vi "Begin.vi"(11 "Image Size":T1=enum."160x120") -> (0 "error out":errorcluster)   [LabVIEW 2012]
doc: "Called before other user functions, this VI is expected to open initial I/O refnums, load in file data, and do all program initialization. Notice that the <B>error out</B> terminal is simply used for data flow. Wiring it to other structures or subVIs ensures that this VI runs first."
uses:
  <vilib>/Rock Robotics/WPI/Camera/WPI_CameraImageSize.ctl
  <vilib>/Rock Robotics/WPI/Camera/WPI_CameraWhite Balance Values.ctl
  <vilib>/Rock Robotics/WPI/Camera/WPI_CameraExposure Values.ctl
  <vilib>/Rock Robotics/WPI/Camera/WPI_CameraFrameRate.ctl
  <vilib>/Rock Robotics/WPI/DriverStation/WPI_DriverStationRobotMode2.ctl
  <vilib>/Rock Robotics/WPI/Joystick/WPI_JoystickDeviceEnum.ctl
  <vilib>/Rock Robotics/SystemInterfaces/DIO/FPGA_DIORelayChannel.ctl
  <vilib>/Rock Robotics/WPI/Relay/WPI_RelayDirection.ctl
  <vilib>/Rock Robotics/SystemInterfaces/DIO/FPGA_DIOChannel.ctl
  <vilib>/Rock Robotics/WPI/Solenoid/WPI_SolenoidChannel.ctl
  <vilib>/Rock Robotics/WPI/Relay/WPI_RelayValue.ctl
  <vilib>/Rock Robotics/SystemInterfaces/DIO/FPGA_DIOPWMChannel.ctl
  <vilib>/Rock Robotics/WPI/SafetyOutput/WPI_SafetyOutputConfigMenu.ctl
  <vilib>/Rock Robotics/SystemInterfaces/AI/FPGA_AIGyroChannel.ctl
  <vilib>/Rock Robotics/SystemInterfaces/AI/FPGA_AIChannel.ctl
  Robot Global Data.vi
  <vilib>/Rock Robotics/WPI/Solenoid/WPI_SolenoidOpenSingle.vi
  <vilib>/Rock Robotics/WPI/MotorControl/WPI_MotorControlOpen Victor.vi
  <vilib>/Rock Robotics/WPI/MotorControl/WPI_MotorControlOpen Jaguar.vi
  <vilib>/Rock Robotics/WPI/RobotDrive/WPI_RobotDriveOpen4MotorWithVictor.vi
  <vilib>/Rock Robotics/WPI/Compressor/WPI_CompressorGetSetRefNum.vi
  <vilib>/Rock Robotics/WPI/RobotDrive/WPI_RobotDriveOpen2MotorWithTalon.vi
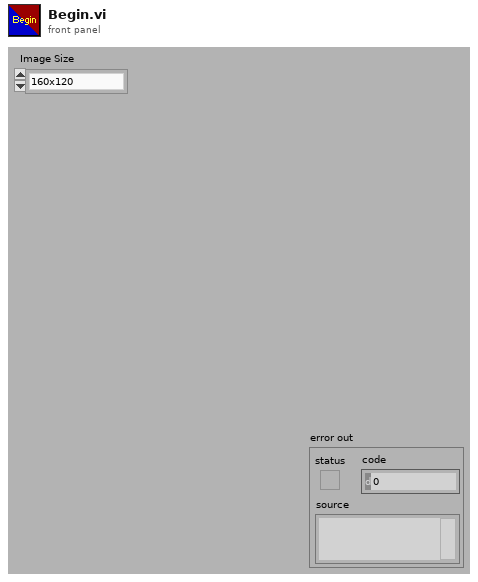
[diagram p1: front panel]
types:
  T1 = typedef "WPI_CameraImageSize.ctl" = enum16{"640x480", "320x240", "160x120"}
  T2 = typedef "WPI_SafetyOutputConfigMenu.ctl" = enum16{"Enable", "Disable"}
  T3 = typedef "WPI_SolenoidChannel.ctl" = enum8{"Solenoid 1", "Solenoid 2", "Solenoid 3", "Solenoid 4", "Solenoid 5", "Solenoid 6", "Solenoid 7", "Solenoid 8", "Invalid"}
  T4 = typedef "FPGA_AIChannel.ctl" = enum8{"AI 1", "AI 2", "AI 3", "AI 4", "AI 5", "AI 6", "AI 7", "AI 8", "Invalid"}
  T5 = typedef "FPGA_DIOPWMChannel.ctl" = enum8{"PWM 1", "PWM 2", "PWM 3", "PWM 4", "PWM 5", "PWM 6", "PWM 7", "PWM 8", "PWM 9", "PWM 10", "Invalid"}
  T6 = typedef "FPGA_AIGyroChannel.ctl" = enum8{"AI 1", "AI 2", "Invalid"}
  T7 = typedef "FPGA_DIOChannel.ctl" = enum8{"DIO 1", "DIO 2", "DIO 3", "DIO 4", "DIO 5", "DIO 6", "DIO 7", "DIO 8", "DIO 9", "DIO 10", "DIO 11", "DIO 12", "DIO 13", "DIO 14", "Invalid"}
  T8 = typedef "WPI_JoystickDeviceEnum.ctl" = enum16{"USB 1", "USB 2", "USB 3", "USB 4", "Kinect 1", "Kinect 2"}
  T9 = typedef "WPI_RelayValue.ctl" = enum16{"Off", "On", "Forward", "Reverse"}
  T10 = typedef "FPGA_DIORelayChannel.ctl" = enum8{"Relay 1", "Relay 2", "Relay 3", "Relay 4", "Relay 5", "Relay 6", "Relay 7", "Relay 8", "Invalid"}
  T11 = typedef "WPI_RelayDirection.ctl" = enum16{"Both directions", "Forward only", "Reverse only"}
  T12 = typedef "WPI_DriverStationRobotMode2.ctl" = enum16{"Autonomous Disabled", "Autonomous Enabled", "Teleop Disabled", "Teleop Enabled", "Timeout", "Finish", "Test Disabled", "Test Enabled"}
  T13 = typedef "WPI_CameraFrameRate.ctl" = u32
  T14 = typedef "WPI_CameraExposure Values.ctl" = enum16{"Auto", "Flicker-free 50 Hz", "Flicker-free 60 Hz", "Hold current"}
  T15 = typedef "WPI_CameraWhite Balance Values.ctl" = enum16{"Auto", "Fixed indoor", "Fixed outdoor 1", "Fixed outdoor 2", "Fixed fluorescent 1", "Fixed fluorescent 2", "Hold current"}
  T16 = typedef "WPI_RobotDriveDevRef.ctl" = cluster{"DevStatus":errorcluster, "Motors[]":T17[], "Square Inputs":bool, "Max Output":dbl, "Isochronous":bool}
  T17 = typedef "WPI_MotorControlDeviceRef.ctl" = cluster{"DeviceStatus":errorcluster, "Type":enum16{"PWM", "CAN"}, "PWM":cluster{"Digital Module":T18, "PWM Channel":T5, "DeadBand":T19}, "CAN":cluster{"Device Number":u8, "Control Mode":T20, "Semaphore":T21, "Max Vout":dbl}, "Invert":bool, "TransformRef":T22, "InvTransformRef":T22}
  T18 = typedef "FPGA_TypedefDigitalModule.ctl" = enum16{"Digital Module 1", "Digital Module 2"}
  T19 = typedef "WPI_PWMDeadband.ctl" = cluster{"Name":string, "maxPositivePwm":i32, "minPositivePwm":i32, "centerPwm":i32, "maxNegativePwm":i32, "minNegativePwm":i32, "angularRange":u16}
  T20 = typedef "WPI_CANJaguar_ControlMode.ctl" = enum8{"Percent VBus", "Current", "Speed", "Position", "Voltage"}
  T21 = typedef "Semaphore RefNum" = refnum<k1>
  T22 = typedef "WPI_PWMTransform_ConPane.ctl" = refnum<vi>
  T23 = typedef "WPI_SolenoidDevRef.ctl" = cluster{"DevStatus":errorcluster, "Solenoid Module":T24, "Forward Solenoid Channel":T3, "Reverse Solenoid Channel":T3}
  T24 = typedef "FPGA_TypedefSolenoidModule.ctl" = enum16{"Solenoid Module 1", "Solenoid Module 2"}
  T25 = typedef "WPI_JoystickDevRef.ctl" = cluster{"Device":T8}
  T26 = typedef "WPI_CameraDevRef.ctl" = cluster{"Camera Address":string, "CameraStatus":errorcluster, "Acquire Image Notifier":refnum<notifier>}
  T27 = typedef "WPI_RelayDevRef.ctl" = cluster{"DevStatus":errorcluster, "Relay Channel":T10, "Digital Module":T18, "Relay Direction":T11}
  T28 = typedef "WPI_GyroDevRef.ctl" = cluster{"DevStatus":errorcluster, "Analog Module":T29, "Analog Channel":T4, "Offset":dbl, "Gain (VoltsPerDegree/Second)":dbl}
  T29 = typedef "FPGA_TypedefAnalogModule.ctl" = enum16{"Analog Module 1", "Analog Module 2"}
  T30 = typedef "WPI_CompressorDevRef.ctl" = cluster{"DevStatus":errorcluster, "DigitalInputDevRef":T31, "RelayDevRef":T27}
  T31 = typedef "WPI_DigitalInputDevRef.ctl" = cluster{"DevStatus":errorcluster, "DIO Channel":T7, "Digital Module":T18}
  T32 = typedef "WPI_AnalogChannelDevRef.ctl" = cluster{"DevStatus":errorcluster, "Analog Module":T29, "Analog Channel":T4}
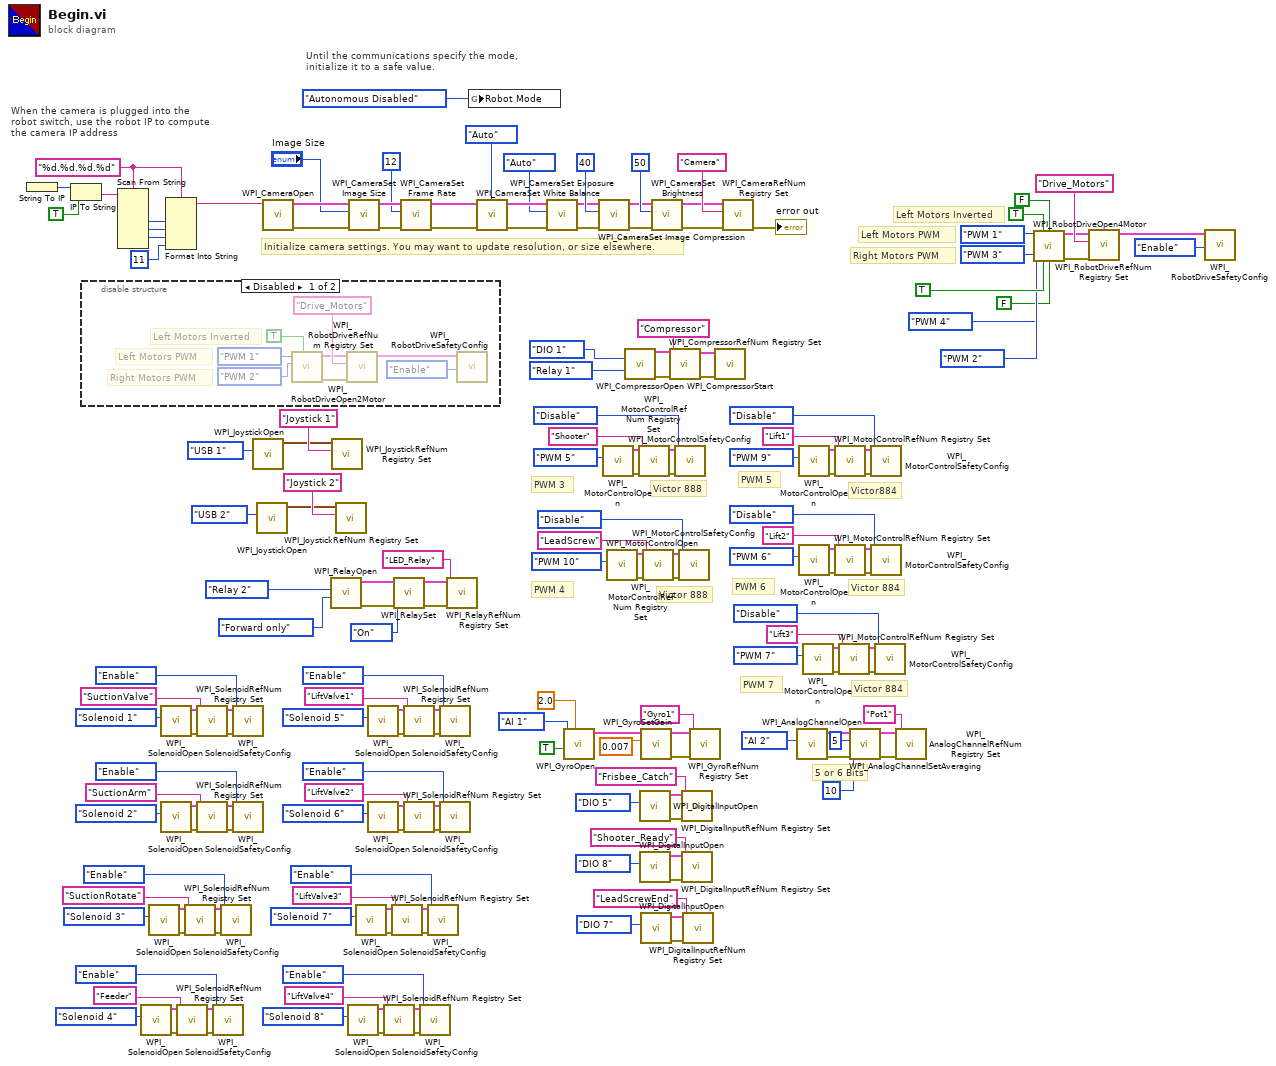
[diagram p0: block diagram]
diagram:
  w38 = "%d.%d.%d.%d" ("format string")
  # "5 or 6 Bits"
  # "PWM 7"
  # "PWM 6"
  # "PWM 5"
  # "PWM 3"
  # "PWM 4"
  # "Right Motors PWM"
  # "Left Motors PWM"
  # "Left Motors Inverted"
  # "Victor884"
  # "Victor 884"
  # "Victor 884"
  # "Victor 888"
  # "Victor 888"
  # "Until the communications specify the mode,\ninitialize it to a safe value."
  # "When the camera is plugged into the\nrobot switch, use the robot IP to compute\nthe camera IP address"
  # "Initialize camera settings. You may want to update resolution, or size elsewhere."
  n1 = String To IP() -> (0:w164:u32)  [unwired: 1 in]
  n2 = IP To String(1:TRUE ("dot notation? (F)"), 2:w164) -> (0:w162:string)
  n3 = disable-structure shown="Disabled" {
    frame Disabled {
      # "Right Motors PWM"
      # "Left Motors PWM"
      # "Left Motors Inverted"
      n4 = call-poly <vilib>:"WPI_RobotDriveOpen2Motor.vi"("Left Motor Inverted"=TRUE, "Right Motor"=FPGA_DIOPWMChannel."PWM 2", "Left Motor"=FPGA_DIOPWMChannel."PWM 1") -> ("error out"=w190:errorcluster, "RobotDriveDevRef"=w189:T16)  [unwired: 7 in]
      n5 = call <vilib>:"WPI_RobotDriveRefNum Registry Set.vi"("error in (no error)"=w190, "refnum name"="Drive_Motors", "RobotDriveDevRef"=w189) -> ("RobotDriveDevRef"=w192:T16)  [unwired: 8 out]
      n6 = call <vilib>:"WPI_RobotDriveSafetyConfig.vi"("mode"=WPI_SafetyOutputConfigMenu."Enable", "RobotDriveDevRef"=w192) -> ()  [unwired: 8 in, 2 out]
    }
    frame Enabled {
    }
  }
  n7 = Scan From String(format string=w38, input string=w162) -> (output 1=w161:i32, output 2=w160:i32, output 3=w159:i32)  [unwired: 7 in, 3 out]
  n8 = call-poly <vilib>:"WPI_SolenoidOpen.vi"("Solenoid Channel"=WPI_SolenoidChannel."Solenoid 4") -> ("error out"=w71:errorcluster, "SolenoidDevRef"=w72:T23)  [unwired: 9 in]
  n9 = call-poly <vilib>:"WPI_SolenoidOpen.vi"("Solenoid Channel"=WPI_SolenoidChannel."Solenoid 3") -> ("error out"=w82:errorcluster, "SolenoidDevRef"=w83:T23)  [unwired: 9 in]
  n10 = call-poly <vilib>:"WPI_SolenoidOpen.vi"("Solenoid Channel"=WPI_SolenoidChannel."Solenoid 1") -> ("error out"=w140:errorcluster, "SolenoidDevRef"=w141:T23)  [unwired: 9 in]
  n11 = call-poly <vilib>:"WPI_SolenoidOpen.vi"("Solenoid Channel"=WPI_SolenoidChannel."Solenoid 2") -> ("error out"=w103:errorcluster, "SolenoidDevRef"=w104:T23)  [unwired: 9 in]
  n12 = Format Into String(format string=w38, w161, w160, w159, 11 ("Compression")) -> (resulting string=w156:string)  [unwired: 2 in, 1 out]
  n13 = call <vilib>:"WPI_SolenoidRefNum Registry Set.vi"("error in (no error)"=w71, "refnum name"="Feeder", "SolenoidDevRef"=w72) -> ("error out"=w68:errorcluster, "SolenoidDevRef"=w67:T23)  [unwired: 7 in]
  n14 = call <vilib>:"WPI_SolenoidRefNum Registry Set.vi"("error in (no error)"=w82, "refnum name"="SuctionRotate", "SolenoidDevRef"=w83) -> ("error out"=w79:errorcluster, "SolenoidDevRef"=w78:T23)  [unwired: 7 in]
  n15 = call <vilib>:"WPI_SolenoidRefNum Registry Set.vi"("error in (no error)"=w140, "refnum name"="SuctionValve", "SolenoidDevRef"=w141) -> ("error out"=w126:errorcluster, "SolenoidDevRef"=w125:T23)  [unwired: 7 in]
  n16 = call <vilib>:"WPI_SolenoidRefNum Registry Set.vi"("error in (no error)"=w103, "refnum name"="SuctionArm", "SolenoidDevRef"=w104) -> ("error out"=w100:errorcluster, "SolenoidDevRef"=w99:T23)  [unwired: 7 in]
  n17 = call <vilib>:"WPI_SolenoidSafetyConfig.vi"("error in (no error)"=w68, "mode"=WPI_SafetyOutputConfigMenu."Enable", "SolenoidDevRef"=w67) -> ()  [unwired: 7 in, 2 out]
  n18 = call <vilib>:"WPI_SolenoidSafetyConfig.vi"("error in (no error)"=w79, "mode"=WPI_SafetyOutputConfigMenu."Enable", "SolenoidDevRef"=w78) -> ()  [unwired: 7 in, 2 out]
  n19 = call <vilib>:"WPI_SolenoidSafetyConfig.vi"("error in (no error)"=w126, "mode"=WPI_SafetyOutputConfigMenu."Enable", "SolenoidDevRef"=w125) -> ()  [unwired: 7 in, 2 out]
  n20 = call <vilib>:"WPI_SolenoidSafetyConfig.vi"("error in (no error)"=w100, "mode"=WPI_SafetyOutputConfigMenu."Enable", "SolenoidDevRef"=w99) -> ()  [unwired: 7 in, 2 out]
  n21 = call <vilib>:"WPI_JoystickOpen.vi"("JoystickDevice"=WPI_JoystickDeviceEnum."USB 1") -> ("JoystickDevRef"=w154:T25)  [unwired: 10 in]
  n22 = call <vilib>:"WPI_JoystickOpen.vi"("JoystickDevice"=WPI_JoystickDeviceEnum."USB 2") -> ("JoystickDevRef"=w64:T25)  [unwired: 10 in]
  n23 = call <vilib>:"WPI_CameraOpen.vi"("Camera Address"=w156) -> ("error out"=w176:errorcluster, "CameraDevRef"=w177:T26)  [unwired: 1 in, 8 out]
  n24 = call <vilib>:"WPI_RelayOpen.vi"("Relay Direction"=WPI_RelayDirection."Forward only", "Relay Channel"=FPGA_DIORelayChannel."Relay 2") -> ("error out"=w137:errorcluster, "RelayDevRef"=w136:T27)  [unwired: 8 in]
  n25 = call <vilib>:"WPI_JoystickRefNum Registry Set.vi"("refnum name"="Joystick 1", "JoystickDevRef"=w154) -> ()  [unwired: 8 in, 2 out]
  n26 = call <vilib>:"WPI_JoystickRefNum Registry Set.vi"("refnum name"="Joystick 2", "JoystickDevRef"=w64) -> ()  [unwired: 8 in, 2 out]
  n27 = call-poly <vilib>:"WPI_SolenoidOpen.vi"("Solenoid Channel"=WPI_SolenoidChannel."Solenoid 8") -> ("error out"=w7:errorcluster, "SolenoidDevRef"=w8:T23)  [unwired: 9 in]
  n28 = call <vilib>:"WPI_CameraSet Image Size.vi"("error in (no error)"=w176, "Image Size"="Image Size", "CameraDevRef"=w177) -> ("error out"=w175:errorcluster, "CameraDevRef Out"=w178:T26)  [unwired: 7 out]
  n29 = call-poly <vilib>:"WPI_SolenoidOpen.vi"("Solenoid Channel"=WPI_SolenoidChannel."Solenoid 7") -> ("error out"=w14:errorcluster, "SolenoidDevRef"=w15:T23)  [unwired: 9 in]
  n30 = call-poly <vilib>:"WPI_SolenoidOpen.vi"("Solenoid Channel"=WPI_SolenoidChannel."Solenoid 5") -> ("error out"=w28:errorcluster, "SolenoidDevRef"=w29:T23)  [unwired: 9 in]
  n31 = call-poly <vilib>:"WPI_SolenoidOpen.vi"("Solenoid Channel"=WPI_SolenoidChannel."Solenoid 6") -> ("error out"=w21:errorcluster, "SolenoidDevRef"=w22:T23)  [unwired: 9 in]
  n32 = call <vilib>:"WPI_SolenoidRefNum Registry Set.vi"("error in (no error)"=w7, "refnum name"="LiftValve4", "SolenoidDevRef"=w8) -> ("error out"=w4:errorcluster, "SolenoidDevRef"=w3:T23)  [unwired: 7 in]
  n33 = call <vilib>:"WPI_SolenoidRefNum Registry Set.vi"("error in (no error)"=w14, "refnum name"="LiftValve3", "SolenoidDevRef"=w15) -> ("error out"=w11:errorcluster, "SolenoidDevRef"=w10:T23)  [unwired: 7 in]
  n34 = call <vilib>:"WPI_RelaySet.vi"("error in (no error)"=w137, "RelayValue"=WPI_RelayValue."On", "RelayDevRef"=w136) -> ("error out"=w134:errorcluster, "RelayDevRef"=w135:T27)  [unwired: 7 in]
  n35 = call <vilib>:"WPI_CameraSet Frame Rate.vi"("error in (no error)"=w175, "Frame Rate (fps)"=T13 12, "CameraDevRef"=w178) -> ("error out"=w174:errorcluster, "CameraDevRef Out"=w180:T26)  [unwired: 7 out]
  n36 = call <vilib>:"WPI_SolenoidRefNum Registry Set.vi"("error in (no error)"=w28, "refnum name"="LiftValve1", "SolenoidDevRef"=w29) -> ("error out"=w25:errorcluster, "SolenoidDevRef"=w24:T23)  [unwired: 7 in]
  n37 = call <vilib>:"WPI_SolenoidRefNum Registry Set.vi"("error in (no error)"=w21, "refnum name"="LiftValve2", "SolenoidDevRef"=w22) -> ("error out"=w18:errorcluster, "SolenoidDevRef"=w17:T23)  [unwired: 7 in]
  n38 = call <vilib>:"WPI_SolenoidSafetyConfig.vi"("error in (no error)"=w4, "mode"=WPI_SafetyOutputConfigMenu."Enable", "SolenoidDevRef"=w3) -> ()  [unwired: 7 in, 2 out]
  n39 = call <vilib>:"WPI_SolenoidSafetyConfig.vi"("error in (no error)"=w11, "mode"=WPI_SafetyOutputConfigMenu."Enable", "SolenoidDevRef"=w10) -> ()  [unwired: 7 in, 2 out]
  n40 = call <vilib>:"WPI_SolenoidSafetyConfig.vi"("error in (no error)"=w25, "mode"=WPI_SafetyOutputConfigMenu."Enable", "SolenoidDevRef"=w24) -> ()  [unwired: 7 in, 2 out]
  n41 = call <vilib>:"WPI_SolenoidSafetyConfig.vi"("error in (no error)"=w18, "mode"=WPI_SafetyOutputConfigMenu."Enable", "SolenoidDevRef"=w17) -> ()  [unwired: 7 in, 2 out]
  n42 = call <vilib>:"WPI_RelayRefNum Registry Set.vi"("error in (no error)"=w134, "refnum name"="LED_Relay", "RelayDevRef"=w135) -> ()  [unwired: 7 in, 2 out]
  n43 = global write "Robot Global Data.vi" "Robot Mode"(WPI_DriverStationRobotMode2."Autonomous Disabled" ("Robot Mode")) -> ()
  n44 = call <vilib>:"WPI_CameraSet White Balance.vi"("error in (no error)"=w174, "White Balance"=WPI_CameraWhite_Balance_Values."Auto", "CameraDevRef"=w180) -> ("error out"=w173:errorcluster, "CameraDevRef Out"=w179:T26)  [unwired: 7 out]
  n45 = call <vilib>:"WPI_CameraSet Exposure.vi"("error in (no error)"=w173, "Exposure"=WPI_CameraExposure_Values."Auto", "CameraDevRef"=w179) -> ("error out"=w172:errorcluster, "CameraDevRef Out"=w182:T26)  [unwired: 7 out]
  n46 = call <vilib>:"WPI_GyroOpen.vi"("Calibration Time (s)"=2.0, "Calibrate On Open"=TRUE, "Analog Channel"=FPGA_AIGyroChannel."AI 1") -> ("GyroDevRef"=w56:T28)  [unwired: 6 in, 2 out]
  n47 = call <vilib>:"WPI_CameraSet Image Compression.vi"("error in (no error)"=w172, "Compression"=40, "CameraDevRef"=w182) -> ("error out"=w171:errorcluster, "CameraDevRef Out"=w181:T26)  [unwired: 7 out]
  n48 = call-poly <vilib>:"WPI_MotorControlOpen.vi"("PWM Channel"=FPGA_DIOPWMChannel."PWM 5") -> ("error out"=w95:errorcluster, "MotorControlDeviceRef"=w96:T17)  [unwired: 9 in]
  n49 = call-poly <vilib>:"WPI_MotorControlOpen.vi"("PWM Channel"=FPGA_DIOPWMChannel."PWM 10") -> ("error out"=w130:errorcluster, "MotorControlDeviceRef"=w131:T17)  [unwired: 9 in]
  n50 = call <vilib>:"WPI_CompressorOpen.vi"("Pressure Switch DIO Channel"=FPGA_DIOChannel."DIO 1", "Relay Channel"=FPGA_DIORelayChannel."Relay 1") -> ("CompressorDevRef"=w145:T30, "error out"=w146:errorcluster)  [unwired: 12 in]
  n51 = call <vilib>:"WPI_MotorControlRefNum Registry Set.vi"("error in (no error)"=w95, "refnum name"="Shooter", "MotorControlDevRef"=w96) -> ("error out"=w93:errorcluster, "MotorControlDevRef"=w92:T17)  [unwired: 7 in]
  n52 = call <vilib>:"WPI_DigitalInputOpen.vi"("DIO Channel"=FPGA_DIOChannel."DIO 5") -> ("error out"=w122:errorcluster, "DigitalInputDevRef"=w121:T31)  [unwired: 9 in]
  n53 = call <vilib>:"WPI_DigitalInputOpen.vi"("DIO Channel"=FPGA_DIOChannel."DIO 8") -> ("error out"=w76:errorcluster, "DigitalInputDevRef"=w75:T31)  [unwired: 9 in]
  n54 = call <vilib>:"WPI_GyroSetGain.vi"("Gain (VoltsPerDegree/Second)"=0.007, "GyroDevRef"=w56) -> ("error out"=w54:errorcluster, "GyroDevRef"=w53:T28)  [unwired: 8 in]
  n55 = call <vilib>:"WPI_DigitalInputOpen.vi"("DIO Channel"=FPGA_DIOChannel."DIO 7") -> ("error out"=w62:errorcluster, "DigitalInputDevRef"=w61:T31)  [unwired: 9 in]
  n56 = call <vilib>:"WPI_MotorControlRefNum Registry Set.vi"("error in (no error)"=w130, "refnum name"="LeadScrew", "MotorControlDevRef"=w131) -> ("error out"=w128:errorcluster, "MotorControlDevRef"=w127:T17)  [unwired: 7 in]
  n57 = call <vilib>:"WPI_CameraSet Brightness.vi"("error in (no error)"=w171, "Brightness"=50, "CameraDevRef"=w181) -> ("error out"=w169:errorcluster, "CameraDevRef Out"=w170:T26)  [unwired: 7 out]
  n58 = call <vilib>:"WPI_CompressorRefNum Registry Set.vi"("error in (no error)"=w146, "refnum name"="Compressor", "CompressorDevRef"=w145) -> ("error out"=w143:errorcluster, "CompressorDevRef"=w142:T30)  [unwired: 7 in]
  n59 = call <vilib>:"WPI_MotorControlSafetyConfig.vi"("error in (no error)"=w93, "mode"=WPI_SafetyOutputConfigMenu."Disable", "MotorControlDevRef"=w92) -> ()  [unwired: 7 in, 2 out]
  n60 = call <vilib>:"WPI_MotorControlSafetyConfig.vi"("error in (no error)"=w128, "mode"=WPI_SafetyOutputConfigMenu."Disable", "MotorControlDevRef"=w127) -> ()  [unwired: 7 in, 2 out]
  n61 = call <vilib>:"WPI_DigitalInputRefNum Registry Set.vi"("error in (no error)"=w122, "refnum name"="Frisbee_Catch", "DigitalInputDevRef"=w121) -> ()  [unwired: 7 in, 2 out]
  n62 = call <vilib>:"WPI_DigitalInputRefNum Registry Set.vi"("error in (no error)"=w76, "refnum name"="Shooter_Ready", "DigitalInputDevRef"=w75) -> ()  [unwired: 7 in, 2 out]
  n63 = call <vilib>:"WPI_DigitalInputRefNum Registry Set.vi"("error in (no error)"=w62, "refnum name"="LeadScrewEnd", "DigitalInputDevRef"=w61) -> ()  [unwired: 7 in, 2 out]
  n64 = call <vilib>:"WPI_GyroRefNum Registry Set.vi"("error in (no error)"=w54, "refnum name"="Gyro1", "GyroDevRef"=w53) -> ()  [unwired: 7 in, 2 out]
  n65 = call <vilib>:"WPI_CompressorStart.vi"("error in (no error)"=w143, "CompressorDevRef"=w142) -> ()  [unwired: 8 in, 2 out]
  n66 = call <vilib>:"WPI_CameraRefNum Registry Set.vi"("error in (no error)"=w169, "refnum name"="Camera", "CameraDevRef"=w170) -> ("error out"=→"error out":errorcluster)  [unwired: 8 out]
  n67 = call <vilib>:"WPI_AnalogChannelOpen.vi"("Analog Channel"=FPGA_AIChannel."AI 2") -> ("error out"=w34:errorcluster, "AIDeviceRef"=w35:T32)  [unwired: 9 in]
  n68 = call-poly <vilib>:"WPI_MotorControlOpen.vi"("PWM Channel"=FPGA_DIOPWMChannel."PWM 9") -> ("error out"=w116:errorcluster, "MotorControlDeviceRef"=w117:T17)  [unwired: 9 in]
  n69 = call-poly <vilib>:"WPI_MotorControlOpen.vi"("PWM Channel"=FPGA_DIOPWMChannel."PWM 6") -> ("error out"=w109:errorcluster, "MotorControlDeviceRef"=w110:T17)  [unwired: 9 in]
  n70 = call-poly <vilib>:"WPI_MotorControlOpen.vi"("PWM Channel"=FPGA_DIOPWMChannel."PWM 7") -> ("error out"=w88:errorcluster, "MotorControlDeviceRef"=w89:T17)  [unwired: 9 in]
  n71 = call <vilib>:"WPI_MotorControlRefNum Registry Set.vi"("error in (no error)"=w116, "refnum name"="Lift1", "MotorControlDevRef"=w117) -> ("error out"=w114:errorcluster, "MotorControlDevRef"=w113:T17)  [unwired: 7 in]
  n72 = call <vilib>:"WPI_MotorControlRefNum Registry Set.vi"("error in (no error)"=w109, "refnum name"="Lift2", "MotorControlDevRef"=w110) -> ("error out"=w107:errorcluster, "MotorControlDevRef"=w106:T17)  [unwired: 7 in]
  n73 = call <vilib>:"WPI_MotorControlRefNum Registry Set.vi"("error in (no error)"=w88, "refnum name"="Lift3", "MotorControlDevRef"=w89) -> ("error out"=w86:errorcluster, "MotorControlDevRef"=w85:T17)  [unwired: 7 in]
  n74 = call <vilib>:"WPI_AnalogChannelSetAveraging.vi"("error in (no error)"=w34, "OversampleBits"=u8 10, "AverageBits"=u8 5, "AIDeviceRef"=w35) -> ("error out"=w33:errorcluster, "AIDeviceRef"=w32:T32)  [unwired: 6 in]
  n75 = call <vilib>:"WPI_MotorControlSafetyConfig.vi"("error in (no error)"=w114, "mode"=WPI_SafetyOutputConfigMenu."Disable", "MotorControlDevRef"=w113) -> ()  [unwired: 7 in, 2 out]
  n76 = call <vilib>:"WPI_MotorControlSafetyConfig.vi"("error in (no error)"=w107, "mode"=WPI_SafetyOutputConfigMenu."Disable", "MotorControlDevRef"=w106) -> ()  [unwired: 7 in, 2 out]
  n77 = call <vilib>:"WPI_MotorControlSafetyConfig.vi"("error in (no error)"=w86, "mode"=WPI_SafetyOutputConfigMenu."Disable", "MotorControlDevRef"=w85) -> ()  [unwired: 7 in, 2 out]
  n78 = call <vilib>:"WPI_AnalogChannelRefNum Registry Set.vi"("error in (no error)"=w33, "refnum name"="Pot1", "AIDeviceRef"=w32) -> ()  [unwired: 7 in, 2 out]
  n79 = call-poly <vilib>:"WPI_RobotDriveOpen4Motor.vi"("Rear Left Motor"=FPGA_DIOPWMChannel."PWM 1" ("Left Motor"), "Rear Left Motor Inverted"=TRUE ("Left Motor Inverted"), "Rear Right Motor Inverted"=FALSE, "Rear Right Motor"=FPGA_DIOPWMChannel."PWM 3" ("Right Motor"), "Front Left Motor"=FPGA_DIOPWMChannel."PWM 4", "Front Right Motor"=FPGA_DIOPWMChannel."PWM 2", "Front Left Motor Inverted"=TRUE, "Front Right Motor Inverted"=FALSE) -> ("RobotDriveDevRef"=w47:T16, "error out"=w48:errorcluster)  [unwired: 6 in]
  n80 = call <vilib>:"WPI_RobotDriveRefNum Registry Set.vi"("error in (no error)"=w48, "refnum name"="Drive_Motors", "RobotDriveDevRef"=w47) -> ("RobotDriveDevRef"=w50:T16)  [unwired: 8 out]
  n81 = call <vilib>:"WPI_RobotDriveSafetyConfig.vi"("mode"=WPI_SafetyOutputConfigMenu."Enable", "RobotDriveDevRef"=w50) -> ()  [unwired: 8 in, 2 out]
